vi "Check_file_header.vi"(0 "Filename":path, 7 "Present Channels only":bool, 9 "Present Channels":string[](array[string]), 11 "Start of read offset (chars.: 0)":i64) -> (3 "File Channels":string[](array[string]), 4 "exists?":bool, 6 "Merged Channels":string[](array[string]), 8 "Start of data (bytes)":i64, 10 "No of bytes/row (approx)":i64, 14 "Current file size (bytes)":i64, 15 "Merged?":bool)   [LabVIEW 2018]
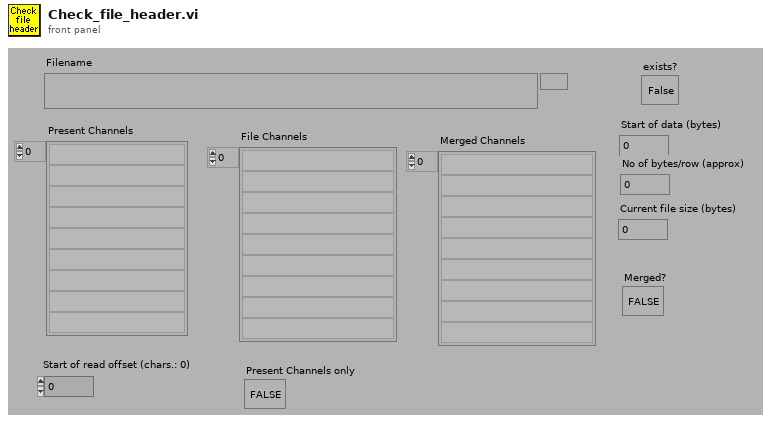
[diagram p1: front panel]
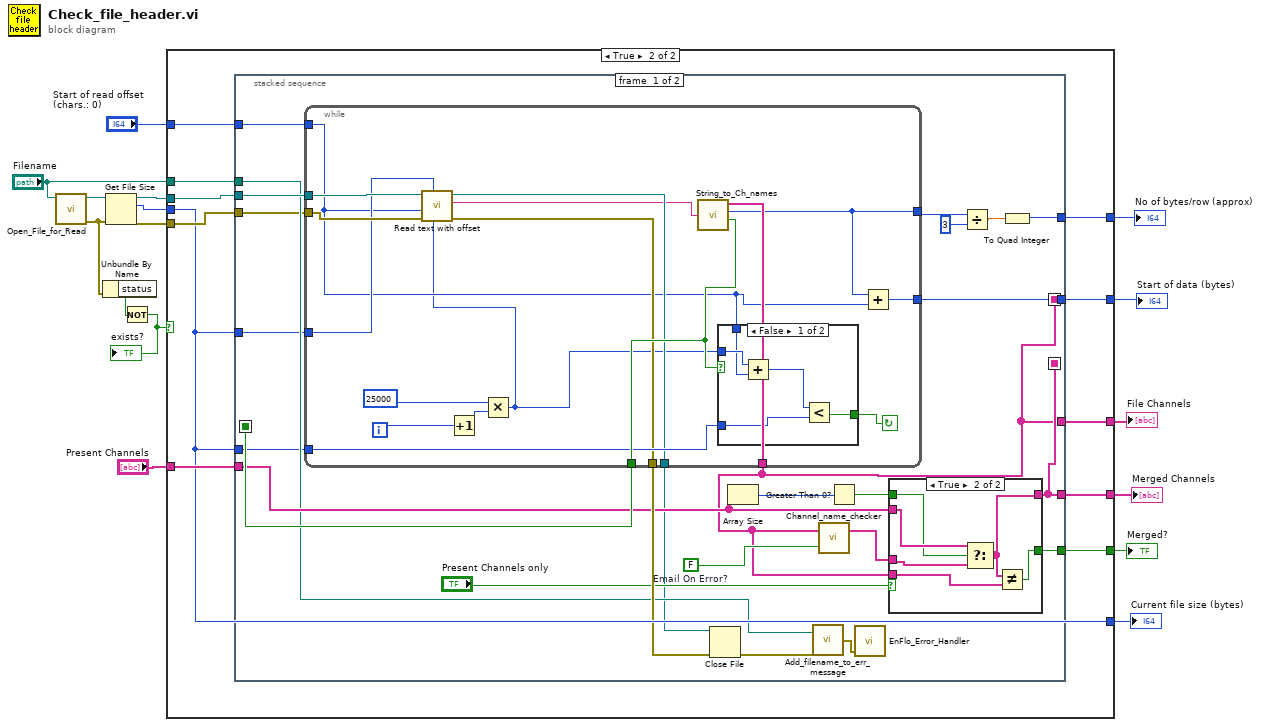
[diagram p0: block diagram]
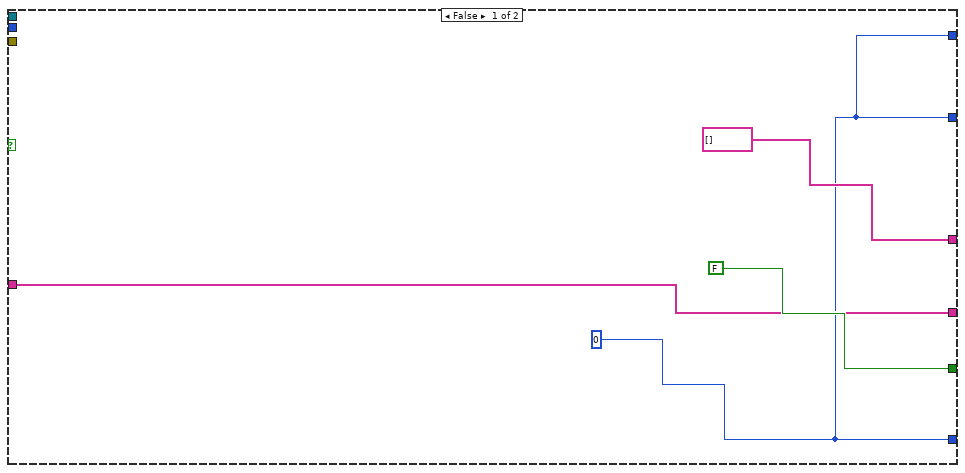
[diagram p2: hidden frame]
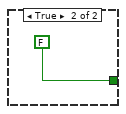
[diagram p3: hidden frame]
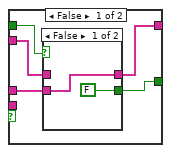
[diagram p4: hidden frame]
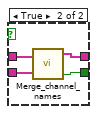
[diagram p5: hidden frame]
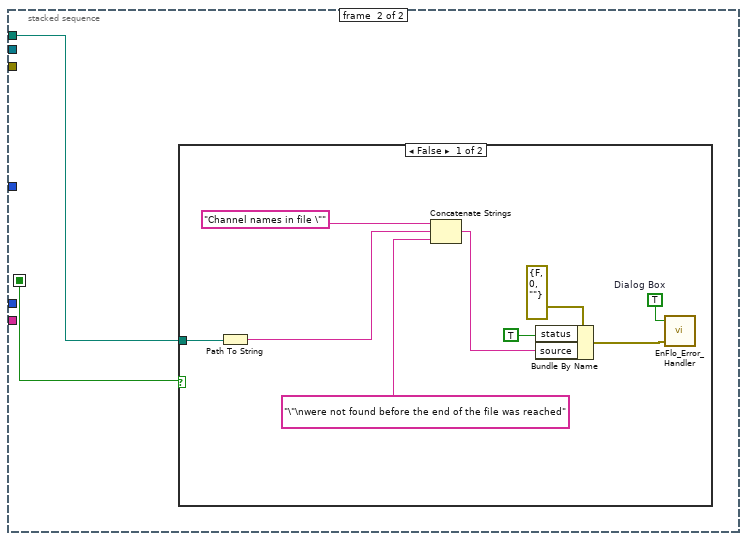
[diagram p6: hidden frame]
diagram:
  n1 = call "Open_File_for_Read.vi"("file path"="Filename") -> ("error out"=w1:errorcluster, "refnum"=w4:refnum<file>)  [unwired: 1 in, 8 out]
  n2 = Unbundle By Name(w1) -> ("status"=w13:bool)
  n3 = Get File Size(file=w4, error in=w1) -> (refnum out=w10:refnum<file>, size (in bytes)=w3:i64, 0:w2:errorcluster)
  n4 = Not(x=w13) -> (.not. x?=w12:bool)
  "exists?" <- w12
  n5 = case shown="True" w12 {
    tunnel: [w18 w30] -> w16
    tunnel: "Present Channels" -> [w18 w31]
    tunnel: [FALSE ("Merged?") w29] -> w14
    tunnel: "Filename" -> [_ w24]
    tunnel: w10 -> [_ w25]
    tunnel: w3 -> [_ w21]
    tunnel: "Start of read offset (chars.: 0)" -> [_ w28]
    tunnel: [w17 w27] -> w8
    tunnel: [w17 w26] -> w7
    tunnel: [w17 w21] -> w6
    tunnel: [string[] [] ("Ch names") w23] -> w5
    tunnel: w2 -> [_ w22]
    frame False {
      w17 = i64 0 ("offset")
    }
    frame True {
      n6 = stacked-sequence {
        seq-local: [w50 _] -> [_ w98]
        seq-local: [w41 _] -> [_ _]
        seq-local: [w43 _] -> [_ _]
        tunnel: w31 -> [w46 _]
        tunnel: [w43 _] -> w30
        tunnel: [w42 _] -> w29
        tunnel: w28 -> [w56 _]
        tunnel: [w34 _] -> w27
        tunnel: [w53 _] -> w26
        tunnel: w25 -> [w51 _]
        tunnel: w24 -> [w38 w97]
        tunnel: [w41 _] -> w23
        tunnel: w22 -> [w37 _]
        tunnel: w21 -> [w33 _]
        tunnel: w21 -> [w32 _]
        frame #0 {
          w48 = FALSE  # Email On Error?
          n7 = while {
            tunnel: [w68] -> w50
            tunnel: [w70] -> w55
            tunnel: w56 -> [w58]
            tunnel: [w62] -> w52
            tunnel: [w72] -> w53
            tunnel: [w73] -> w41
            tunnel: w51 -> [w63]
            tunnel: w37 -> [w64]
            tunnel: [w61] -> w36
            tunnel: w33 -> [w66]
            tunnel: w32 -> [w59]
            i -> [w69]
            stop <- w67 continue-if-true
            n8 = Increment(x=w69) -> (x+1=w71:i32)
            n9 = Multiply(x=25000 ("count"), y=w71) -> (x*y=w57:i32)
            n10 = call "Read text with offset.vi"("Count"=w57, "File Size"=w59, "Error In"=w64, "Start of read offset (chars.: 0)"=w58, "Refnum In"=w63) -> ("Error out"=w62:errorcluster, "text"=w60:string, "refnum out"=w61:refnum<file>)  [unwired: 3 in, 1 out]
            n11 = call "String_to_Ch_names.vi"("Spreadsheet string"=w60) -> ("Ch names"=w73:string[], "Title length (Bytes)"=w70:i32, "Title Rows Found?"=w68:bool)  [unwired: 1 out]
            n12 = case shown="False" w68 {
              tunnel: [w74 FALSE] -> w67
              tunnel: w57 -> [w77 _]
              tunnel: w66 -> [w78 _]
              tunnel: w58 -> [w76 _]
              frame False {
                n13 = Add(x=w77, y=w76) -> (x+y=w75:i64)
                n14 = Less?(x=w75, y=w78) -> (x < y?=w74:bool)
              }
              frame True {
              }
            }
            n15 = Add(x=w70, y=w58) -> (x+y=w72:i64)
          }
          n16 = Close File(refnum=w36, error in=w52) -> (error out=w40:errorcluster)  [unwired: 1 out]
          n17 = Array Size(array=w46) -> (size(s)=w47:i32)
          n18 = call "Add_filename_to_err_message.vi"("error in (no error)"=w40, "Path"=w38) -> ("error out"=w39:errorcluster)
          n19 = call "Channel_name_checker.vi"("Email On Error?"=w48, "Channel names"=w41) -> ("Channel names Out"=w44:string[])  [unwired: 1 out]
          n20 = Greater Than 0?(x=w47) -> (x > 0?=w45:bool)
          n21 = call "EnFlo_Error_Handler.vi"("error in (no error)"=w39) -> ()  [unwired: 2 in, 3 out]
          n22 = case shown="True" "Present Channels only" {
            tunnel: w46 -> [w84 w96]
            tunnel: [w83 w93] -> w43
            tunnel: w44 -> [w82 w94]
            tunnel: w45 -> [w81 w95]
            tunnel: [w80 w91] -> w42
            tunnel: w41 -> [_ w92]
            frame False {
              n23 = case shown="False" w81 {
                tunnel: w84 -> [_ w90]
                tunnel: [w86 w89] -> w83
                tunnel: [FALSE ("Merged?") w88] -> w80
                tunnel: w82 -> [w86 w87]
                frame False {
                }
                frame True {
                  n24 = call "Merge_channel_names.vi"("Preferred Channel array"=w90, "Channel array"=w87) -> ("Merged Channels"=w89:string[], "Channel Array Changed?"=w88:bool)  [unwired: 1 out]
                }
              }
            }
            frame True {
              n25 = Select(t=w96, s=w95, f=w94) -> (s? t:f=w93:string[])
              n26 = Not Equal?(x=w93, y=w92) -> (x != y?=w91:bool)
            }
          }
          n27 = Divide(x=w55, y=3) -> (x/y=w35:dbl)
          n28 = To Quad Integer(1:w35) -> (0:w34:i64)
        }
        frame #1 {
          n29 = case shown="False" w98 {
            tunnel: w97 -> [w105 _]
            frame False {
              w102 = TRUE  # Dialog Box
              n30 = Path To String(path=w105) -> (string=w104:string)
              n31 = Concatenate Strings("Channel names in file \"" ("message"), w104, "\"\nwere not found before the end of the file was reached" ("message")) -> (w100:string)
              n32 = Bundle By Name(cluster=errorcluster {"status"=FALSE, "code"=0, "source"=""} ("error in (no error)"), "status"=TRUE ("Bundle Element"), "source"=w100) -> (w99:errorcluster)
              n33 = call "EnFlo_Error_Handler.vi"("error in (no error)"=w99, "Dialog Box (T)"=w102) -> ()  [unwired: 1 in, 3 out]
            }
            frame True {
            }
          }
        }
      }
    }
  }
  "Merged?" <- w14
  "Merged Channels" <- w16
  "Current file size (bytes)" <- w6
  "Start of data (bytes)" <- w7
  "No of bytes/row (approx)" <- w8
  "File Channels" <- w5
